vi "Read WaitingTest.vi"(8 "error in (no error)":errorcluster, 11 "TestSeqClass in":refnum<class "TestSeqClass.lvclass">) -> (0 "error out":errorcluster, 2 "WaitingTestSeq":refnum<notifier>, 3 "TestSeqClass out":refnum<class "TestSeqClass.lvclass">)   [LabVIEW 2017, in "TestSeqClass.lvclass"]
uses:
  TestSeqClass.lvclass
  Typedef/TestSeqType.ctl
  TestMeasureStep/TestMeasureStep.lvclass
  TestSeqClass.lvclass/TestSeqClass.ctl
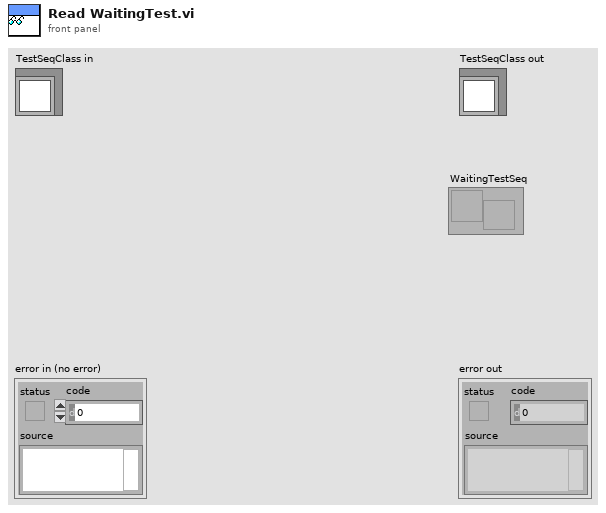
[diagram p1: front panel]
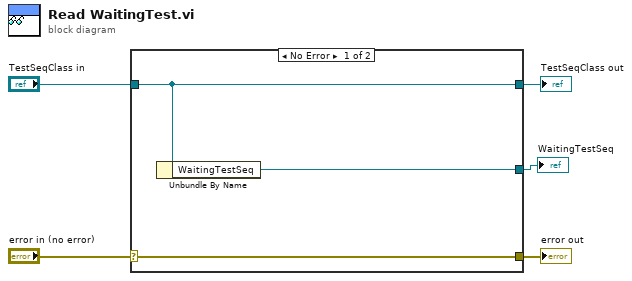
[diagram p0: block diagram]
diagram:
  n1 = case shown="No Error" "error in (no error)" {
    selector: "error in (no error)" -> [w8 w9]
    tunnel: [w8 w9] -> w4
    tunnel: [w7 w10] -> w2
    tunnel: "TestSeqClass in" -> [w7 w10]
    tunnel: [w6 _] -> w1
    frame No Error {
      n2 = Unbundle By Name(w7) -> ("WaitingTestSeq"=w6:refnum<notifier>)
    }
    frame Error {
    }
  }
  "error out" <- w4
  "TestSeqClass out" <- w2
  "WaitingTestSeq" <- w1
